vi "ma_sml_Calculating Filter Power Spectrum.vi"(7 "adjacent channel specifications":cluster{"offset":dbl, "bandwidth":dbl}[](array[cluster]), 8 "filter info":T3[](array[typedef]) {"filter type" items=["None", "RRC"]}, 9 "spectral info":T4 {"window" items=["Rectangle"=0, "Hanning"=1, "Hamming"=2, "Blackman-Harris"=3, "Exact Blackman"=4, "Blackman"=5, "Flat Top"=6, "4 Term B-Harris "=7, "7 Term B-Harris"=8, "Low Sidelobe"=9, "Blackman Nuttall"=11, "Triangle"=30, "Bartlett-Hanning"=31, "Bohman"=32, "Parzen"=33, "Welch"=34, "Kaiser"=60, "Dolph-Chebyshev"=61, "Gaussian"=62]}, 10 "spectrum properties":T2={"f0"=0.0, "df"=1.0, "#spectral lines"=0} {"df" format="%.2f"; "f0" format="%.2f"}, 11 "center channel specification":cluster{"center frequency":dbl, "bandwidth":dbl}) -> (3 "filtered power spectrum":T1 {"spectrum" format="%.2f"; "df" format="%.2f"; "f0" format="%.2f"})   [LabVIEW 2020, in "NI_MAPro.lvlib"]
uses:
  NI_MAPro.lvlib
  ma_sml_Spectral Info.ctl
  ma_sml_Filter Info.ctl
  ma_sml_Spectrum Cluster (real).ctl
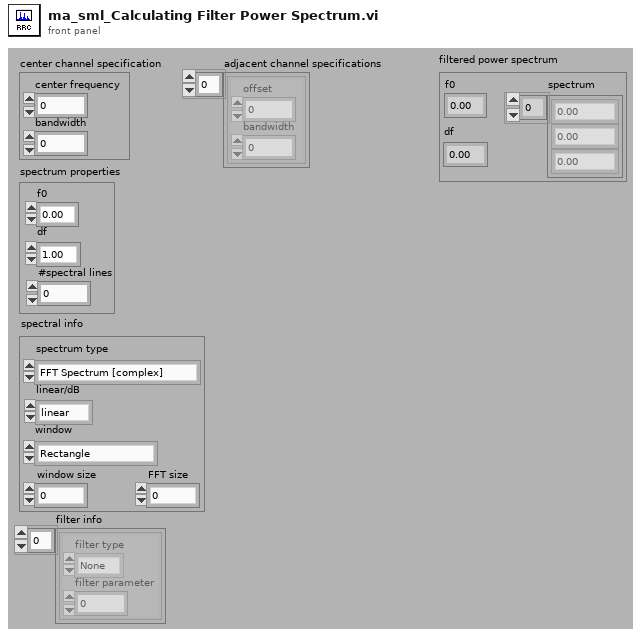
[diagram p1: front panel]
types:
  T1 = typedef "NI_MAPro.lvlib/ma_sml_Spectrum Cluster (real).ctl" = cluster{"f0":dbl, "df":dbl, "spectrum":dbl[]}
  T2 = cluster{"f0":dbl, "df":dbl, "#spectral lines":i32}
  T3 = typedef "NI_MAPro.lvlib/ma_sml_Filter Info.ctl" = cluster{"filter type":u16, "filter parameter":dbl}
  T4 = typedef "NI_MAPro.lvlib/ma_sml_Spectral Info.ctl" = cluster{"spectrum type":enum16{"FFT Spectrum [complex]", "Amplitude [Magnitude]", "Power [Magnitude^2]", "Cross Spectrum [complex]", "Frequency Response [Complex]"}, "linear/dB":enum16{"linear", "dB"}, "window":u16, "window size":i32, "FFT size":i32}
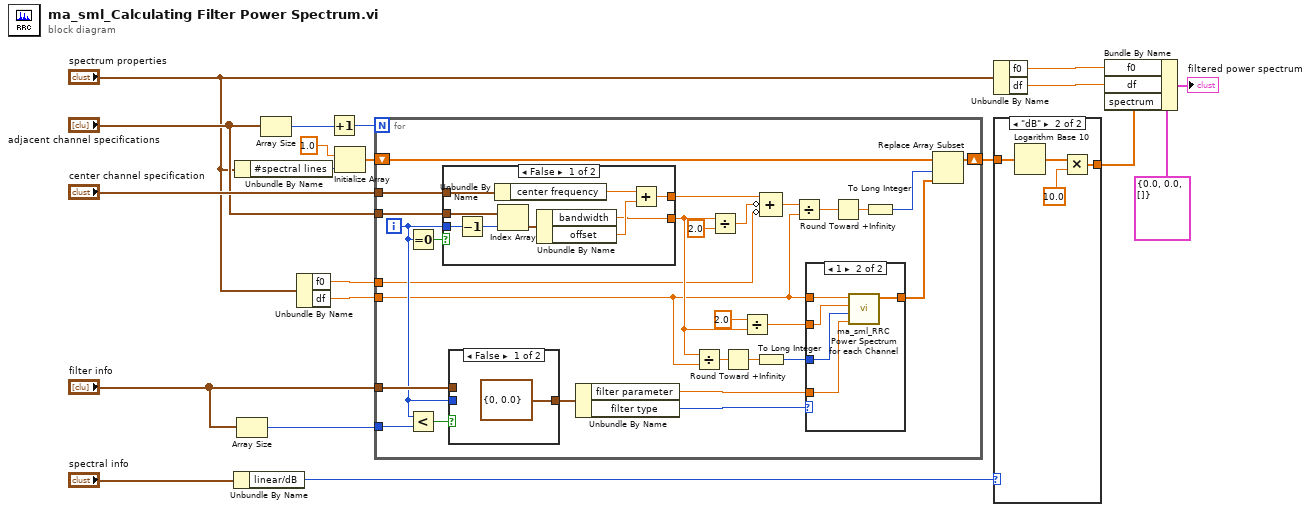
[diagram p0: block diagram]
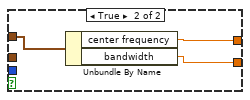
[diagram p2: hidden frame]
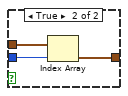
[diagram p3: hidden frame]
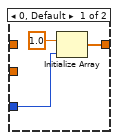
[diagram p4: hidden frame]
diagram:
  n1 = Unbundle By Name("spectral info") -> ("linear/dB"=w13:enum16{"linear", "dB"})
  n2 = Unbundle By Name("spectrum properties") -> ("#spectral lines"=w10:i32)
  n3 = Array Size(array="filter info") -> (size(s)=w17:i32)
  n4 = Array Size(array="adjacent channel specifications") -> (size(s)=w12:i32)
  n5 = Unbundle By Name("spectrum properties") -> ("f0"=w2:dbl, "df"=w1:dbl)
  n6 = Increment(x=w12) -> (x+1=w11:i32)
  n7 = Initialize Array(1.0 ("element"), w10) -> (w15:dbl[])
  n8 = for {
    N: w11 -> [_]
    tunnel: "filter info" -> [w38]
    tunnel: w17 -> [w35]
    shift-right: [w32] -> w14
    shift-left: w15 -> [w33]
    tunnel: "center channel specification" -> [w30]
    tunnel: "adjacent channel specifications" -> [w29]
    tunnel: w2 -> [w22]
    tunnel: w1 -> [w21]
    i -> [w28]
    n9 = Equal To 0?(x=w28) -> (x = 0?=w31:bool)
    n10 = Less?(x=w28, y=w35) -> (x < y?=w36:bool)
    n11 = case shown="False" w31 {
      tunnel: [w49 w58] -> w25
      tunnel: w30 -> [w57 w60]
      tunnel: [w50 w59] -> w34
      tunnel: w29 -> [w56 _]
      tunnel: w28 -> [w54 _]
      frame False {
        n12 = Decrement(x=w54) -> (x-1=w55:i32)
        n13 = Unbundle By Name(w57) -> ("center frequency"=w52:dbl)
        n14 = Index Array(array=w56, index=w55) -> (element=w53:cluster{"offset":dbl, "bandwidth":dbl})
        n15 = Unbundle By Name(w53) -> ("bandwidth"=w49:dbl, "offset"=w51:dbl)
        n16 = Add(x=w52, y=w51) -> (x+y=w50:dbl)
      }
      frame True {
        n17 = Unbundle By Name(w60) -> ("center frequency"=w59:dbl, "bandwidth"=w58:dbl)
      }
    }
    n18 = case shown="False" w36 {
      tunnel: w38 -> [_ w64]
      tunnel: w28 -> [_ w63]
      tunnel: [T3 {"filter type"=0, "filter parameter"=0.0} ("element") w62] -> w37
      frame False {
      }
      frame True {
        n19 = Index Array(array=w64, index=w63) -> (element=w62:T3)
      }
    }
    n20 = Unbundle By Name(w37) -> ("filter parameter"=w40:dbl, "filter type"=w39:u16)
    n21 = Divide(x=w25, y=w21) -> (x/y=w48:dbl)
    n22 = Divide(x=w25, y=2.0) -> (x/y=w26:dbl)
    n23 = Round Toward +Infinity(x=w48) -> (ceil(x): smallest int >= x=w47:dbl)
    n24 = Divide(x=2.0 ("y"), y=w25) -> (x/y=w23:dbl)
    n25 = To Long Integer(number=w47) -> (32bit integer=w46:i32)
    n26 = Compound Arithmetic op=ADD(w34, invert w26, invert w22) -> (w45:dbl)
    n27 = Divide(x=w45, y=w21) -> (x/y=w43:dbl)
    n28 = case shown="1" w39 {
      tunnel: w46 -> [w66 w69]
      tunnel: w23 -> [_ w70]
      tunnel: w40 -> [_ w68]
      tunnel: w21 -> [_ w71]
      tunnel: [w65 w72] -> w41
      frame 0, Default {
        n29 = Initialize Array(1.0 ("element"), w66) -> (w65:dbl[])
      }
      frame 1 {
        n30 = call "ma_sml_RRC Power Spectrum for each Channel.vi"("beta"=w68, "n"=w69, "T"=w70, "df"=w71) -> ("RRC power spectrum"=w72:dbl[])  [unwired: 7 in]
      }
    }
    n31 = Round Toward +Infinity(x=w43) -> (ceil(x): smallest int >= x=w44:dbl)
    n32 = To Long Integer(number=w44) -> (32bit integer=w42:i32)
    n33 = Replace Array Subset(array=w33, new element=w41, index=w42) -> (w32:dbl[])
  }
  n34 = Unbundle By Name("spectrum properties") -> ("f0"=w8:dbl, "df"=w7:dbl)
  n35 = case shown="\"dB\"" w13 {
    tunnel: w14 -> [w73 w77]
    tunnel: [w73 w76] -> w9
    frame "linear", Default {
    }
    frame "dB" {
      n36 = Logarithm Base 10(1:w77) -> (0:w74:dbl[])
      n37 = Multiply(x=w74, y=10.0) -> (x*y=w76:dbl[])
    }
  }
  n38 = Bundle By Name(cluster=T1 {"f0"=0.0, "df"=0.0, "spectrum"=[]} ("filtered power spectrum"), "f0"=w8, "df"=w7, "spectrum"=w9) -> (→"filtered power spectrum":T1)
